vi "forlooptunnel.vi"() -> ()   [LabVIEW 2021]
panel:
  out "Numeric":i32
  out "Array 2":i32[](array[numeric])
  out "Array":i32[](array[numeric])
  out "x+1":i32
  out "Count":i32
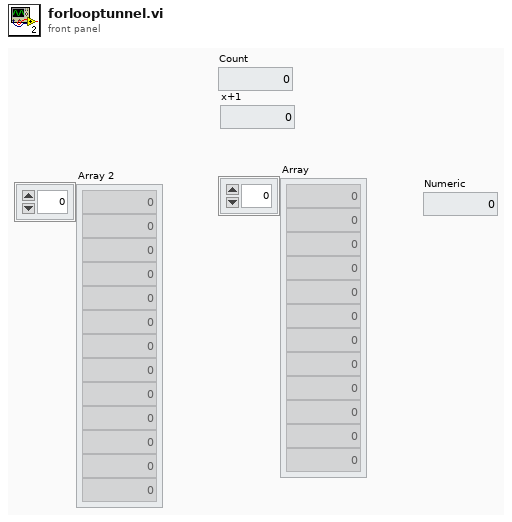
[diagram p1: front panel]
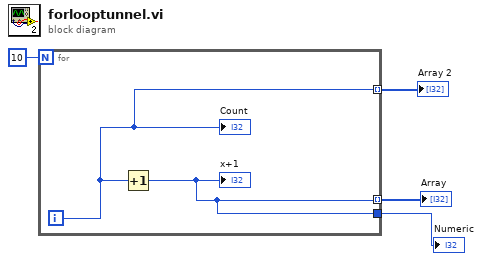
[diagram p0: block diagram]
diagram:
  n1 = for {
    N: 10 -> [_]
    tunnel: [w5] -> w3 mode=indexing
    tunnel: [w6] -> w2 mode=indexing
    tunnel: [w5] -> w1
    i -> [w6]
    n2 = Increment(x=w6) -> (x+1=w5:i32)
    "x+1" <- w5
    "Count" <- w6
  }
  "Array" <- w3
  "Array 2" <- w2
  "Numeric" <- w1
